vi "WMI Reboot.vi"(8 "error in":errorcluster, 11 "Method":enum16{"Reboot", "Shutdown"}(ring)) -> (0 "error out":errorcluster)   [LabVIEW 2013]
doc: "This VI calls the method <b>Reboot</b> in the class <b>Win32_OperatingSystem</b> to reboot the Windows machine. Prior to the call, we set <b>ConnectionOptions.EnablePrivileges</b> to TRUE in order to not get the 'Privilege not held' exception."
uses:
  System.Management
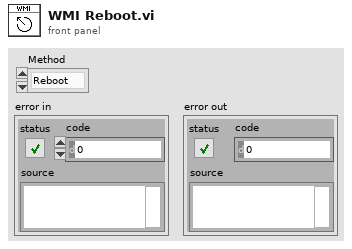
[diagram p1: front panel]
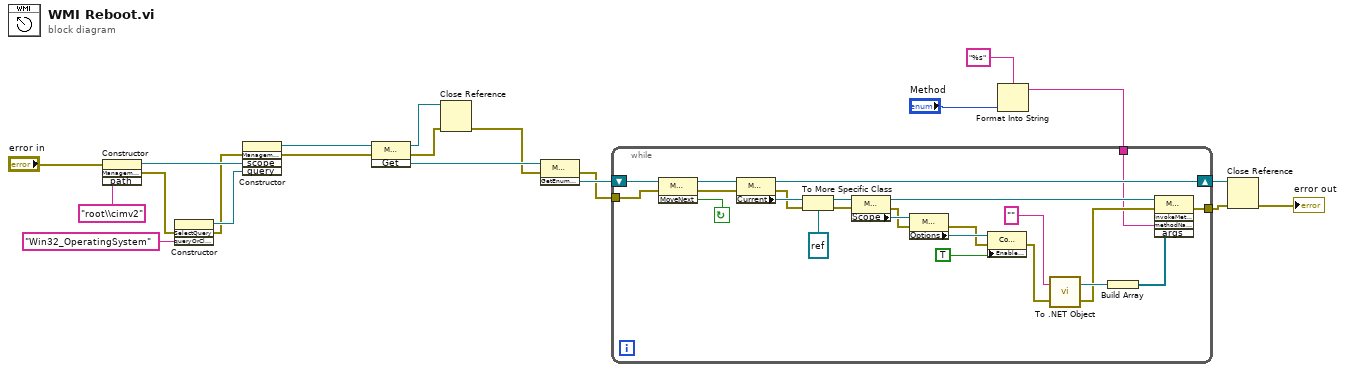
[diagram p0: block diagram]
diagram:
  n1 = constructor class="ManagementScope"(error in="error in", "path"="root\\cimv2" ("Scope")) -> (reference out=w19:refnum<k24>, error out=w8:errorcluster)  [unwired: 2 in, 2 out]
  n2 = constructor class="SelectQuery"(error in=w8, "queryOrClassName"="Win32_OperatingSystem") -> (reference out=w18:refnum<k24>, error out=w7:errorcluster)  [unwired: 2 in, 2 out]
  n3 = constructor class="ManagementObjectSearcher"(error in=w7, "scope"=w19, "query"=w18) -> (reference out=w9:refnum<k24>, error out=w15:errorcluster)  [unwired: 2 in, 3 out]
  n4 = invoke class="ManagementObjectSearcher" method="Get"(reference=w9, error in=w15) -> (reference out=w13:refnum<k24>, error out=w12:errorcluster, "Get"=w17:refnum<k24>)  [unwired: 1 in]
  n5 = Close Reference(reference=w13, error in (no error)=w12) -> (error out=w11:errorcluster)
  n6 = invoke class="ManagementObjectCollection" method="GetEnumerator"(reference=w17, error in=w11) -> (error out=w14:errorcluster, "GetEnumerator"=w16:refnum<k24>)  [unwired: 1 in, 1 out]
  n7 = Format Into String(format string="%s", "Method") -> (resulting string=w1:string)  [unwired: 2 in, 1 out]
  n8 = while {
    shift-right: [w41] -> w10
    shift-left: w16 -> [w45]
    tunnel: w14 -> [w38]
    tunnel: [w35] -> w6
    tunnel: w1 -> [w22]
    stop <- w44 continue-if-true
    n9 = invoke class="ManagementObjectCollection+Mana" method="MoveNext"(reference=w45, error in=w38) -> (reference out=w42:refnum<k24>, error out=w37:errorcluster, "MoveNext"=w44:bool)  [unwired: 1 in]
    n10 = property class="ManagementObjectCollection+Mana"(reference=w42, error in=w37) -> (reference out=w41:refnum<k24>, error out=w39:errorcluster, "Current"=w40:refnum<k24>)
    n11 = To More Specific Class(target class=refnum<k24> refnum ("Current"), reference=w40, error in=w39) -> (specific class reference=w36:refnum<k24>, error out=w34:errorcluster)
    n12 = property class="ManagementObject"(reference=w36, error in=w34) -> (reference out=w26:refnum<k24>, error out=w27:errorcluster, "Scope"=w30:refnum<k24>)
    n13 = property class="ManagementScope"(reference=w30, error in=w27) -> (error out=w25:errorcluster, "Options"=w29:refnum<k24>)  [unwired: 1 out]
    n14 = property class="ConnectionOptions"(reference=w29, error in=w25, "EnablePrivileges"=TRUE) -> (error out=w24:errorcluster)  [unwired: 1 out]
    n15 = call <vilib>:"To .NET Object.vi"("error in (no error)"=w24, "anything"="" ("methodName")) -> ("error out"=w23:errorcluster, ".NET object"=w32:refnum<k24>)
    n16 = Build Array(w32) -> (w31:refnum<k24>[])
    n17 = invoke class="ManagementObject" method="InvokeMethod"(reference=w26, error in=w23, "methodName"=w22, "args"=w31) -> (error out=w35:errorcluster)  [unwired: 1 in, 4 out]
  }
  n18 = Close Reference(reference=w10, error in (no error)=w6) -> (error out=→"error out":errorcluster)
